vi "From JSON Text (DBL).vi"(7 "Data Type (default value)":dbl, 9 "error in (no error)":errorcluster, 10 "Offset":i32, 11 "JSON":string) -> (1 "error out":errorcluster, 2 "Offset past match":i32, 3 "Number":dbl format="%#.6f")   [LabVIEW 2020, in "JSONtext.lvlib"]
doc: "Convert the JSON Value at Offset into a LabVIEW type."
uses:
  <vilib>/JDP Science/JSONtext/JSONtext.lvlib
  <vilib>/JDP Science/JSONtext/support/Get DBL.vi
  <vilib>/JDP Science/JSONtext/support/Get Number Text.vi
  <vilib>/JDP Science/JSONtext/String Subset.vi
  <vilib>/JDP Science/JSONtext/Parsing/Advance past Number.vi
  <vilib>/JDP Science/JSONtext/Parsing/Parsing Error in converting to LabVIEW type.vi
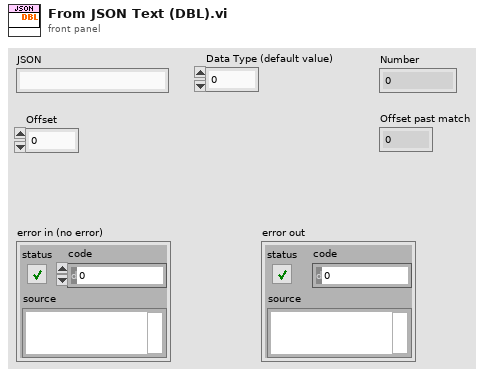
[diagram p1: front panel]
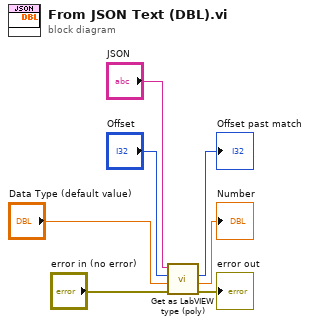
[diagram p0: block diagram]
diagram:
  n1 = call-poly <vilib>:"Get as LabVIEW type (poly).vi"("error in (no error)"="error in (no error)", "Data Type (default value)"="Data Type (default value)", "Offset"="Offset", "JSON"="JSON") -> ("error out"=→"error out":errorcluster, "Number"=→"Number":dbl, "Offset past match"=→"Offset past match":i32)  [unwired: 5 in]
